vi "Get Connections for Inputs.vi"(8 "error in (no error)":errorcluster, 9 "Inputs":dbl[](array[numeric]), 10 "States Changed":bool[](array[boolean]), 11 "Routing Channel Configurations":T1[](array[typedef])) -> (0 "error out":errorcluster, 3 "Compiled Connections Indices":i32[](array[numeric]))   [LabVIEW 2017, in "Routing and Faulting Engine.lvlib"]
uses:
  Routing and Faulting Engine.lvlib
  Shared/Routing Channel Configuration.ctl
  Shared/Value-Connections Map.ctl
  Shared/Routing and Faulting Shared.lvlib
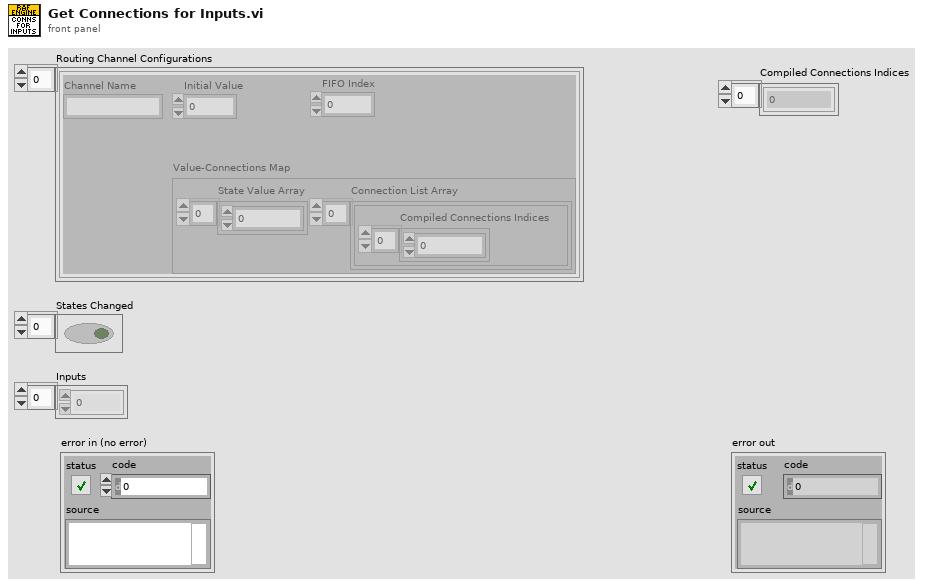
[diagram p1: front panel]
types:
  T1 = typedef "Routing and Faulting Shared.lvlib/Routing Channel Configuration.ctl" = cluster{"Channel Name":string, "Initial Value":dbl, "FIFO Index":i32, "Value-Connections Map":T2}
  T2 = typedef "Routing and Faulting Shared.lvlib/Value-Connections Map.ctl" = cluster{"State Value Array":i32[], "Connection List Array":cluster{"Compiled Connections Indices":i32[]}[]}
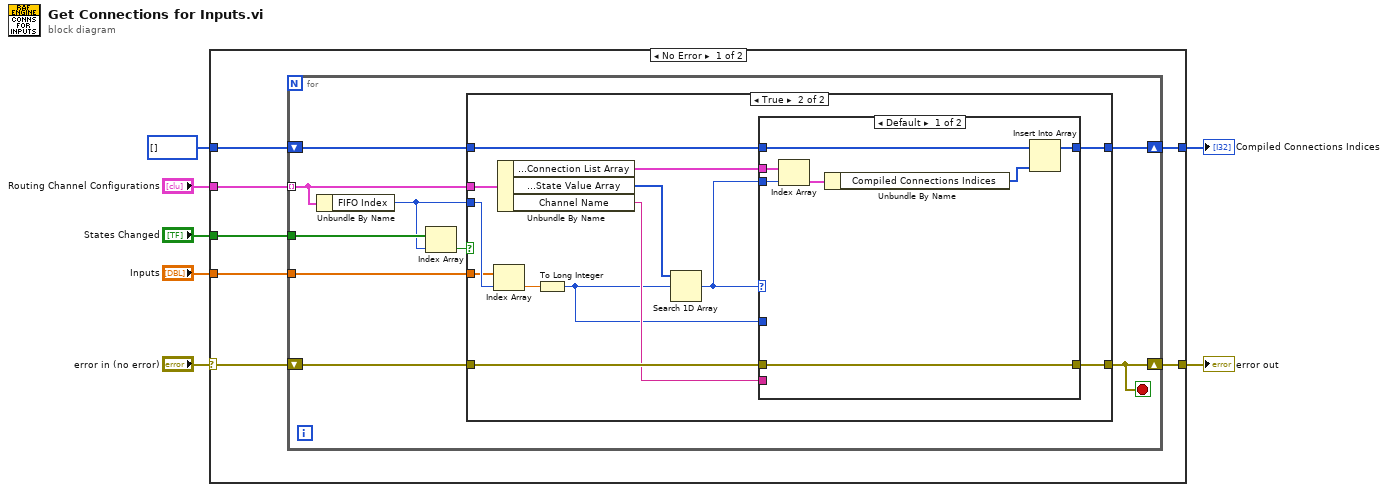
[diagram p0: block diagram]
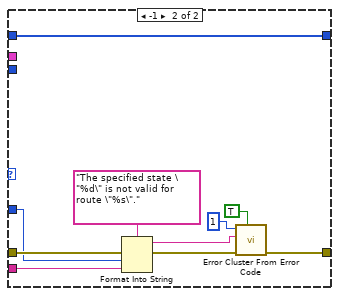
[diagram p3: hidden frame]
diagram:
  n1 = case shown="No Error" "error in (no error)" {
    selector: "error in (no error)" -> [w11 w57]
    tunnel: "Inputs" -> [w14 _]
    tunnel: "States Changed" -> [w13 _]
    tunnel: "Routing Channel Configurations" -> [w12 _]
    tunnel: [w10 w57] -> w3
    tunnel: [w9 w56] -> w2
    tunnel: i32[] [] -> [w8 w56]
    frame No Error {
      n2 = for {
        tunnel: w13 -> [w22]
        tunnel: w12 -> [w23] mode=indexing
        tunnel: w14 -> [w20]
        shift-right: [w17] -> w10
        shift-left: w11 -> [w18]
        shift-right: [w15] -> w9
        shift-left: w8 -> [w16]
        stop <- w17 stop-if-true
        n3 = Unbundle By Name(w23) -> ("FIFO Index"=w19:i32)
        n4 = Index Array(array=w22, index=w19) -> (element=w21:bool)
        n5 = case shown="True" w21 {
          tunnel: w23 -> [_ w38]
          tunnel: w20 -> [_ w36]
          tunnel: w19 -> [_ w37]
          tunnel: w18 -> [w25 w33]
          tunnel: [w25 w32] -> w17
          tunnel: w16 -> [w24 w27]
          tunnel: [w24 w26] -> w15
          frame False {
            # "State didn't change. No connections."
          }
          frame True {
            n6 = Index Array(array=w36, index=w37) -> (element=w35:dbl)
            n7 = Unbundle By Name(w38) -> ("Value-Connections Map.Connection List Array"=w28:cluster{"Compiled Connections Indices":i32[]}[], "Value-Connections Map.State Value Array"=w34:i32[], "Channel Name"=w31:string)
            n8 = To Long Integer(number=w35) -> (32bit integer=w30:i32)
            n9 = Search 1D Array(1D array=w34, element=w30) -> (index of element=w29:i32)  [unwired: 1 in]
            n10 = case shown="Default" w29 {
              tunnel: w33 -> [w45 w51]
              tunnel: [w45 w55] -> w32
              tunnel: w31 -> [_ w49]
              tunnel: w30 -> [_ w48]
              tunnel: w29 -> [w43 _]
              tunnel: w28 -> [w42 _]
              tunnel: w27 -> [w41 w46]
              tunnel: [w40 w46] -> w26
              frame Default {
                n11 = Index Array(array=w42, index=w43) -> (element=w44:cluster{"Compiled Connections Indices":i32[]})
                n12 = Unbundle By Name(w44) -> ("Compiled Connections Indices"=w39:i32[])
                n13 = Insert Into Array(array=w41, new element=w39) -> (w40:i32[])  [unwired: 1 in]
              }
              frame -1 {
                n14 = Format Into String(format string="The specified state \"%d\" is not valid for route \"%s\".", error in=w51, w48, w49) -> (resulting string=w50:string, error out=w52:errorcluster)  [unwired: 1 in]
                n15 = call <vilib>:"Error Cluster From Error Code.vi"("show call chain? (False)"=TRUE, "error in (no error)"=w52, "error message (\"\")"=w50, "error code (0)"=1) -> ("error out"=w55:errorcluster)  [unwired: 5 in]
              }
            }
          }
        }
      }
    }
    frame Error {
    }
  }
  "error out" <- w3
  "Compiled Connections Indices" <- w2
